vi "禹山叶绿素a校准.vi"() -> ()   [LabVIEW 2016, in "斯坦道多参数.lvlib"]
uses:
  <vilib>/Utility/miscctls.llb/LVPointTypeDef.ctl
  <vilib>/Analysis/NI_AALBase.lvlib
  <vilib>/Analysis/NI_AALPro.lvlib
  <vilib>/Utility/config.llb/NI_LVConfig.lvlib
panel:
  out "滤波设定":dbl
  out "通讯状态":string
  out "第二点校准值":dbl
  out "第一点校准值":dbl
  out "最小值":sgl format="%.2g"
  out "最大值":sgl format="%.2g"
  in  "校准停止":bool
  in  "校准模式":u16(ring) items=["两点校准", "单点校准"]
  in  "标液2":dbl
  in  "标液1":dbl
  out "波形图表":sgl(graph) caption="历史曲线"
  out "温度测量值":dbl caption="温度" format="%#.2f"
  out "变异系数":dbl format="%.6g"
  out "standard deviation":dbl caption="标准差" format="%0.2f"
  out "mean":dbl caption="均值" format="%0.2f"
  out "提示":string
  in  "校准启动":bool
  out "测试值":dbl format="%#.2f"
  out "电极斜率":dbl format="%#.6f"
  out "电极零点":dbl format="%#.6f"
  # "叶绿素a电极设定"
  # "请选择校准模式:"
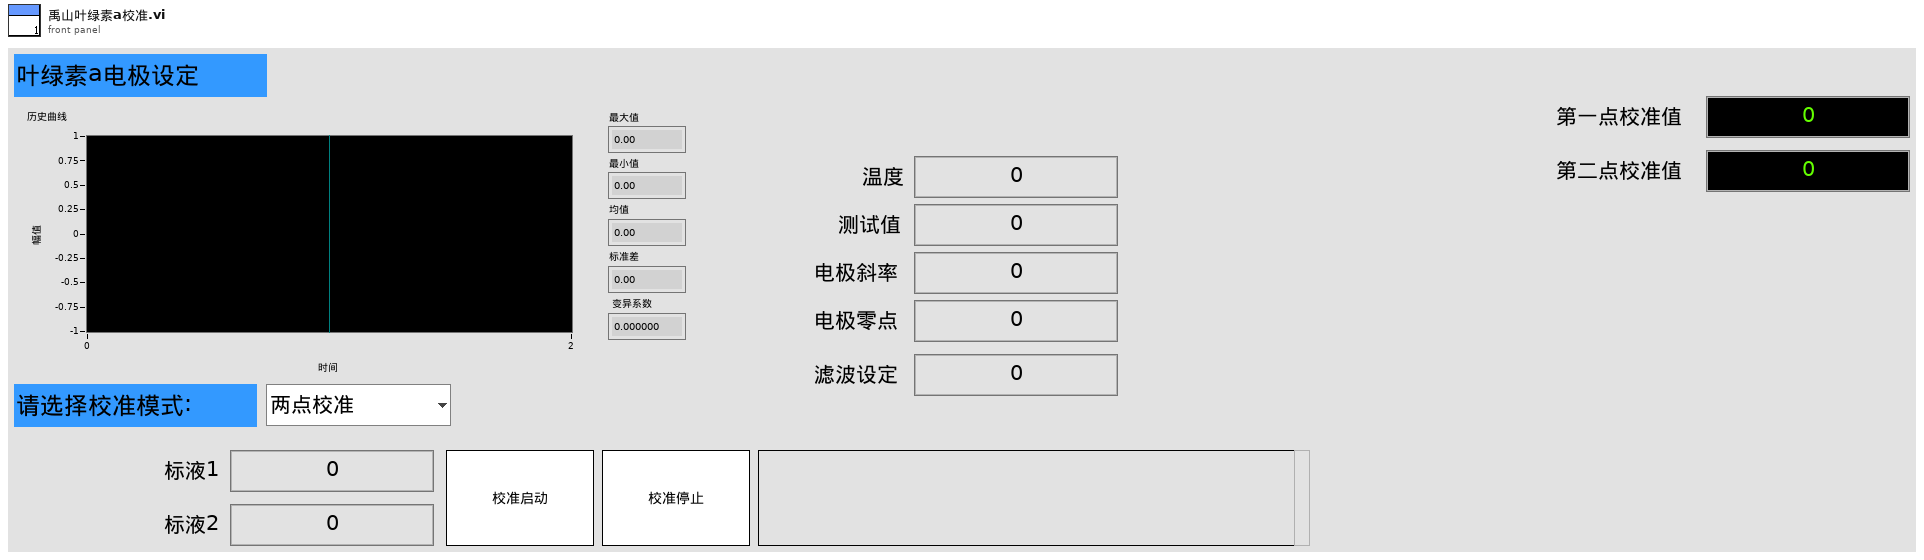
[diagram p1: front panel]
types:
  T1 = enum16{"pH", "DO", "Cond", "Turb", "ORP", "叶绿素a", "藻密度"}
  T2 = typedef "LVPointTypeDef.ctl" = cluster{"Horizontal":i16, "Vertical":i16}
  T3 = cluster{"pH":u32, "DO":u32, "Cond":u32, "Turb":u32, "叶绿素a":u32, "藻密度":u32, "ORP":u32}
  T4 = typedef "NI_LVConfig.lvlib/Config Data RefNum.ctl" = refnum<k1>
  T5 = enum8{"Enabled", "Disabled", "Disabled and Grayed Out"}
  T6 = cluster{"ph":bool, "DO":bool, "Cond":bool, "Turb":bool, "叶绿素a":bool, "藻密度":bool, "ORP":bool}
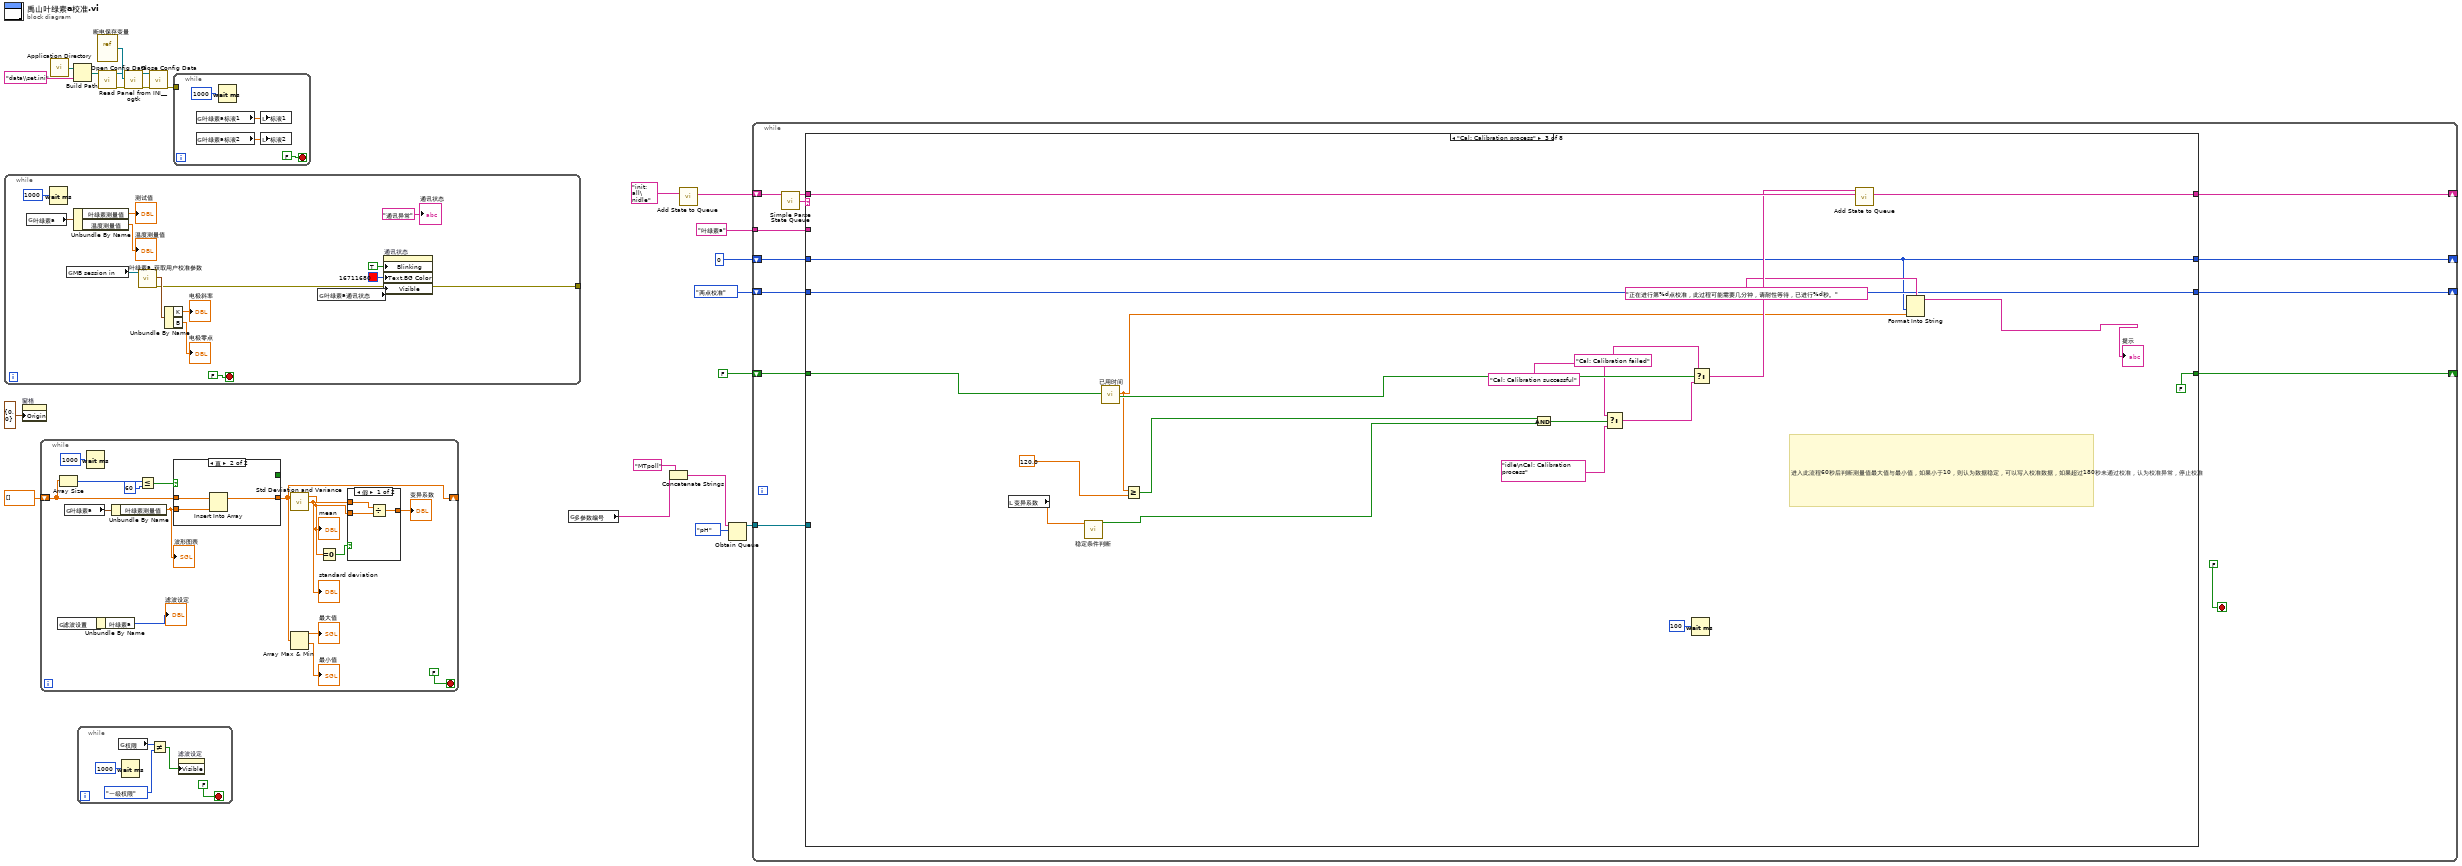
[diagram p0: block diagram]
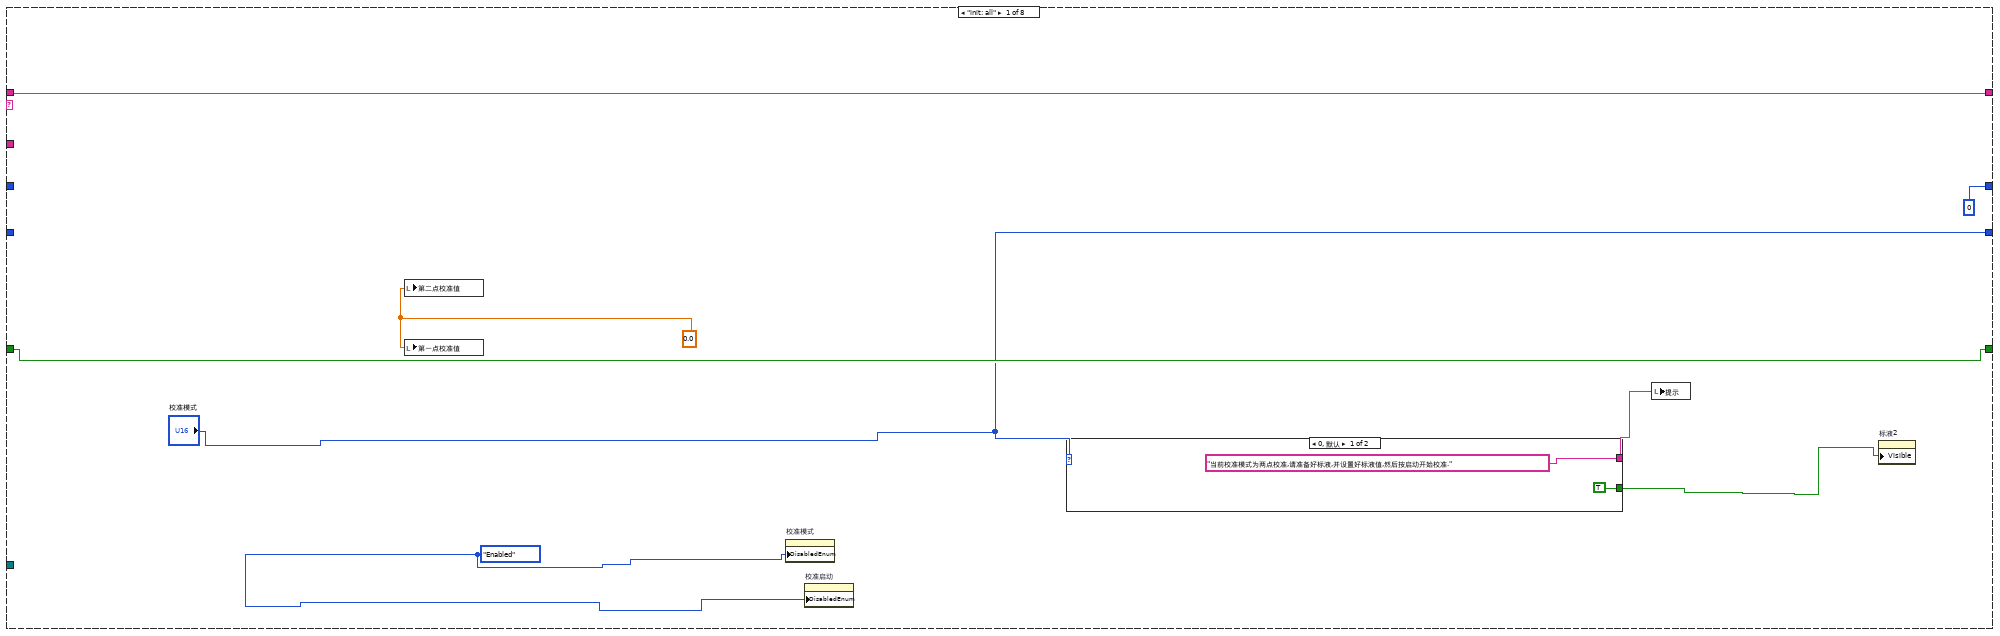
[diagram p2: hidden frame]
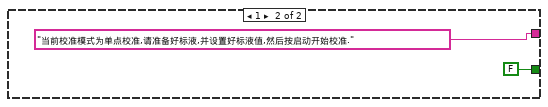
[diagram p3: hidden frame]
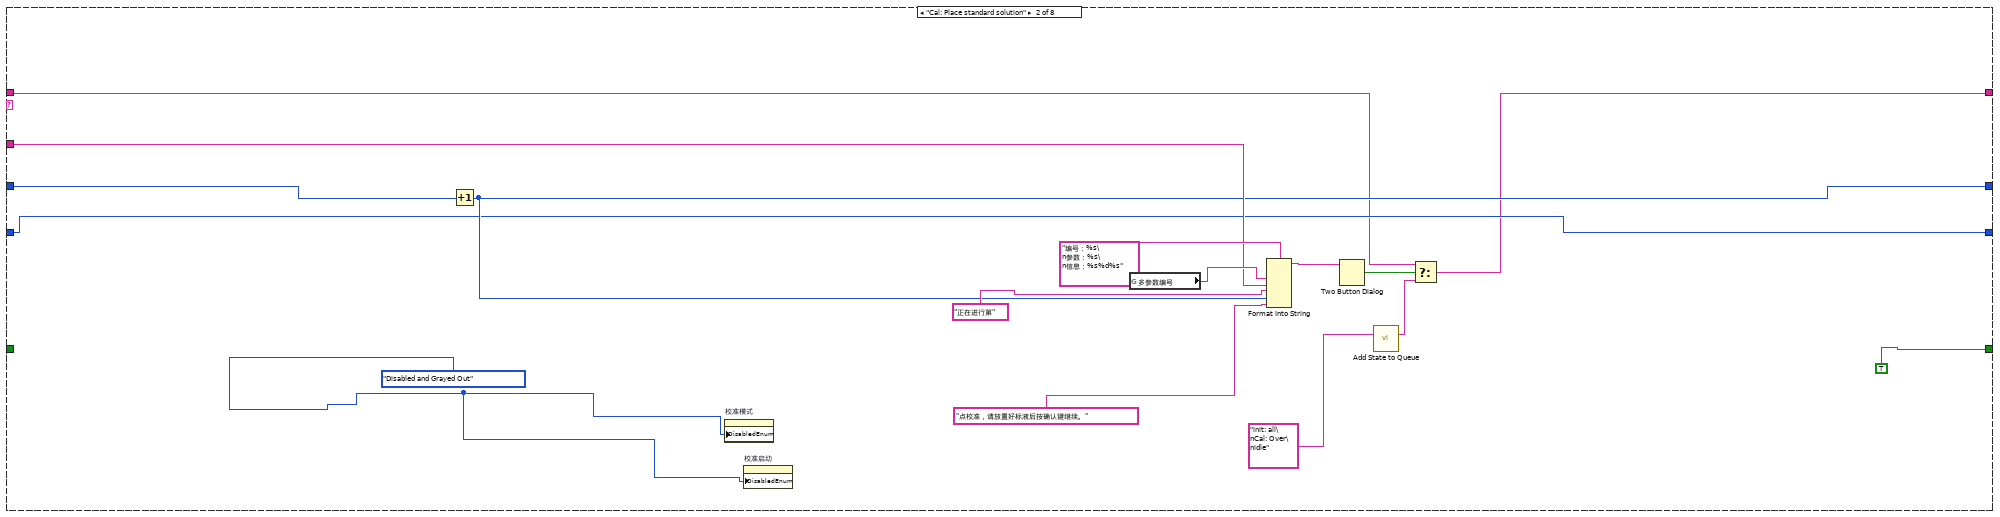
[diagram p4: hidden frame]
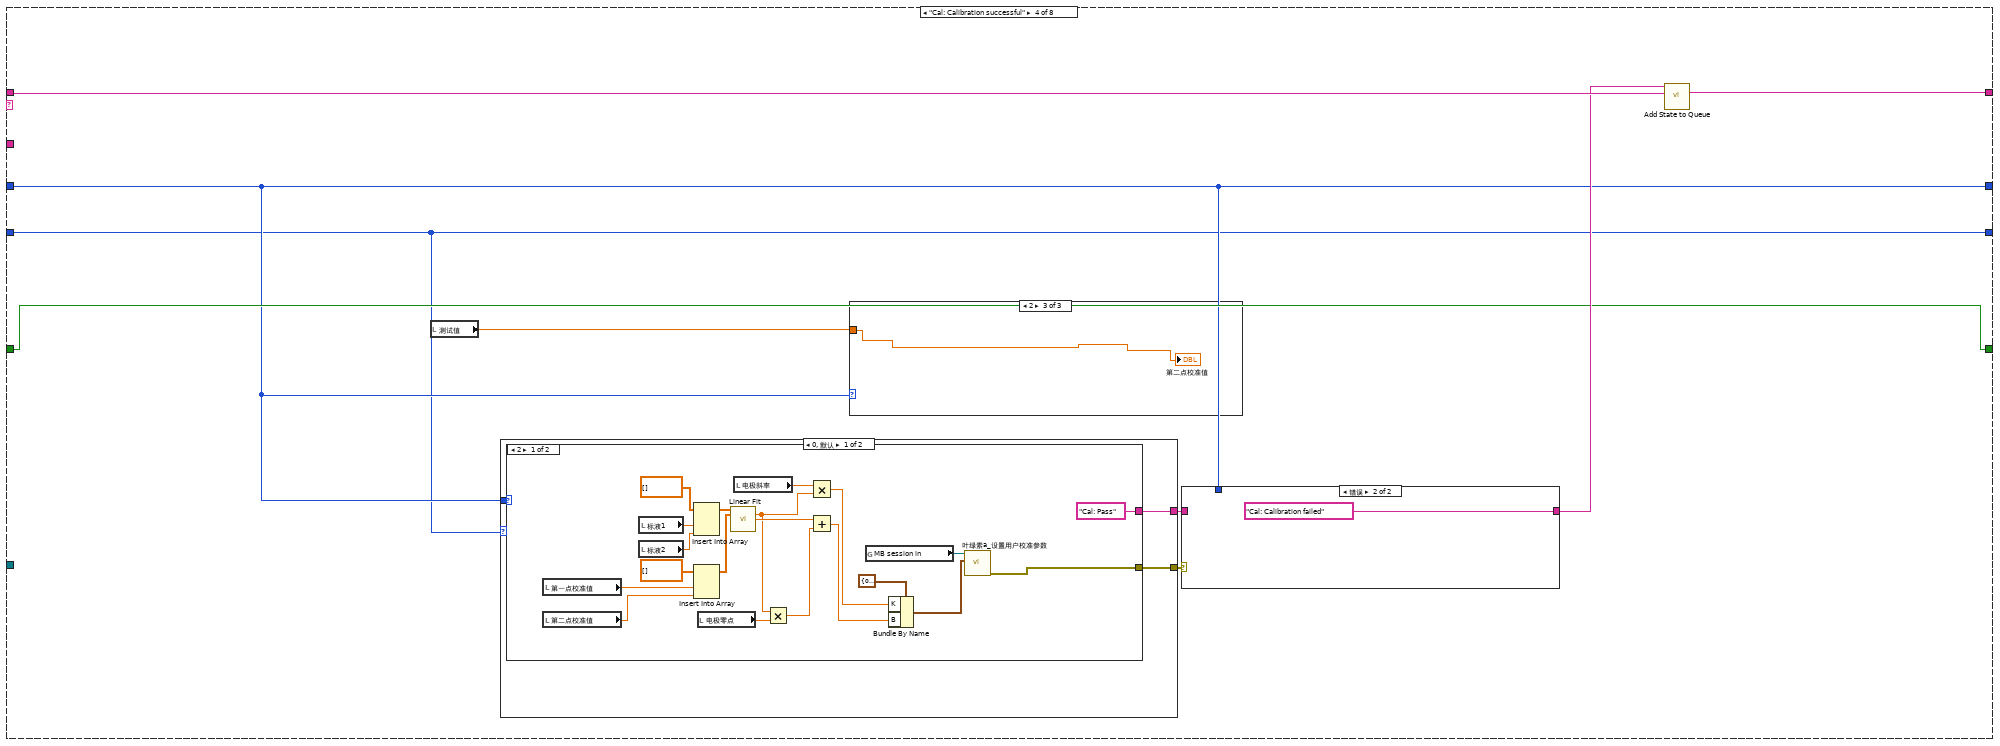
[diagram p5: hidden frame]
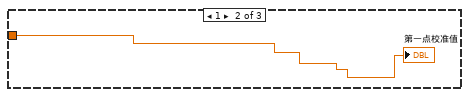
[diagram p7: hidden frame]
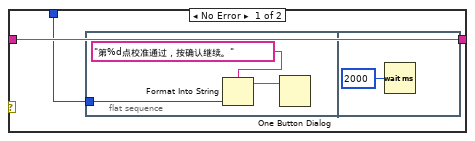
[diagram p8: hidden frame]
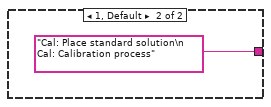
[diagram p9: hidden frame]
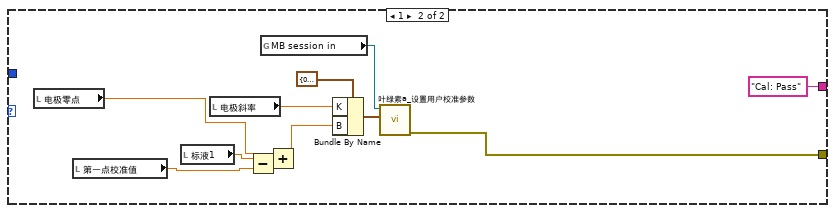
[diagram p10: hidden frame]
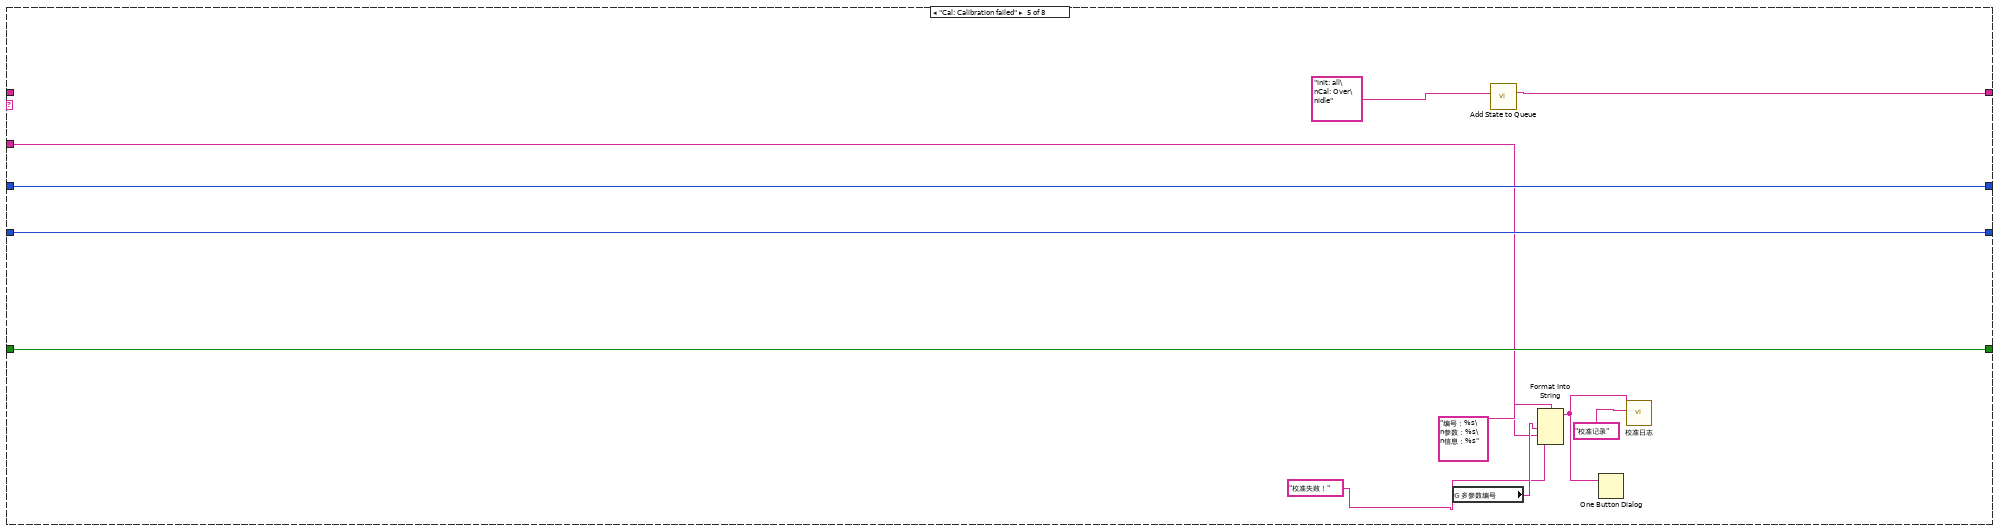
[diagram p11: hidden frame]
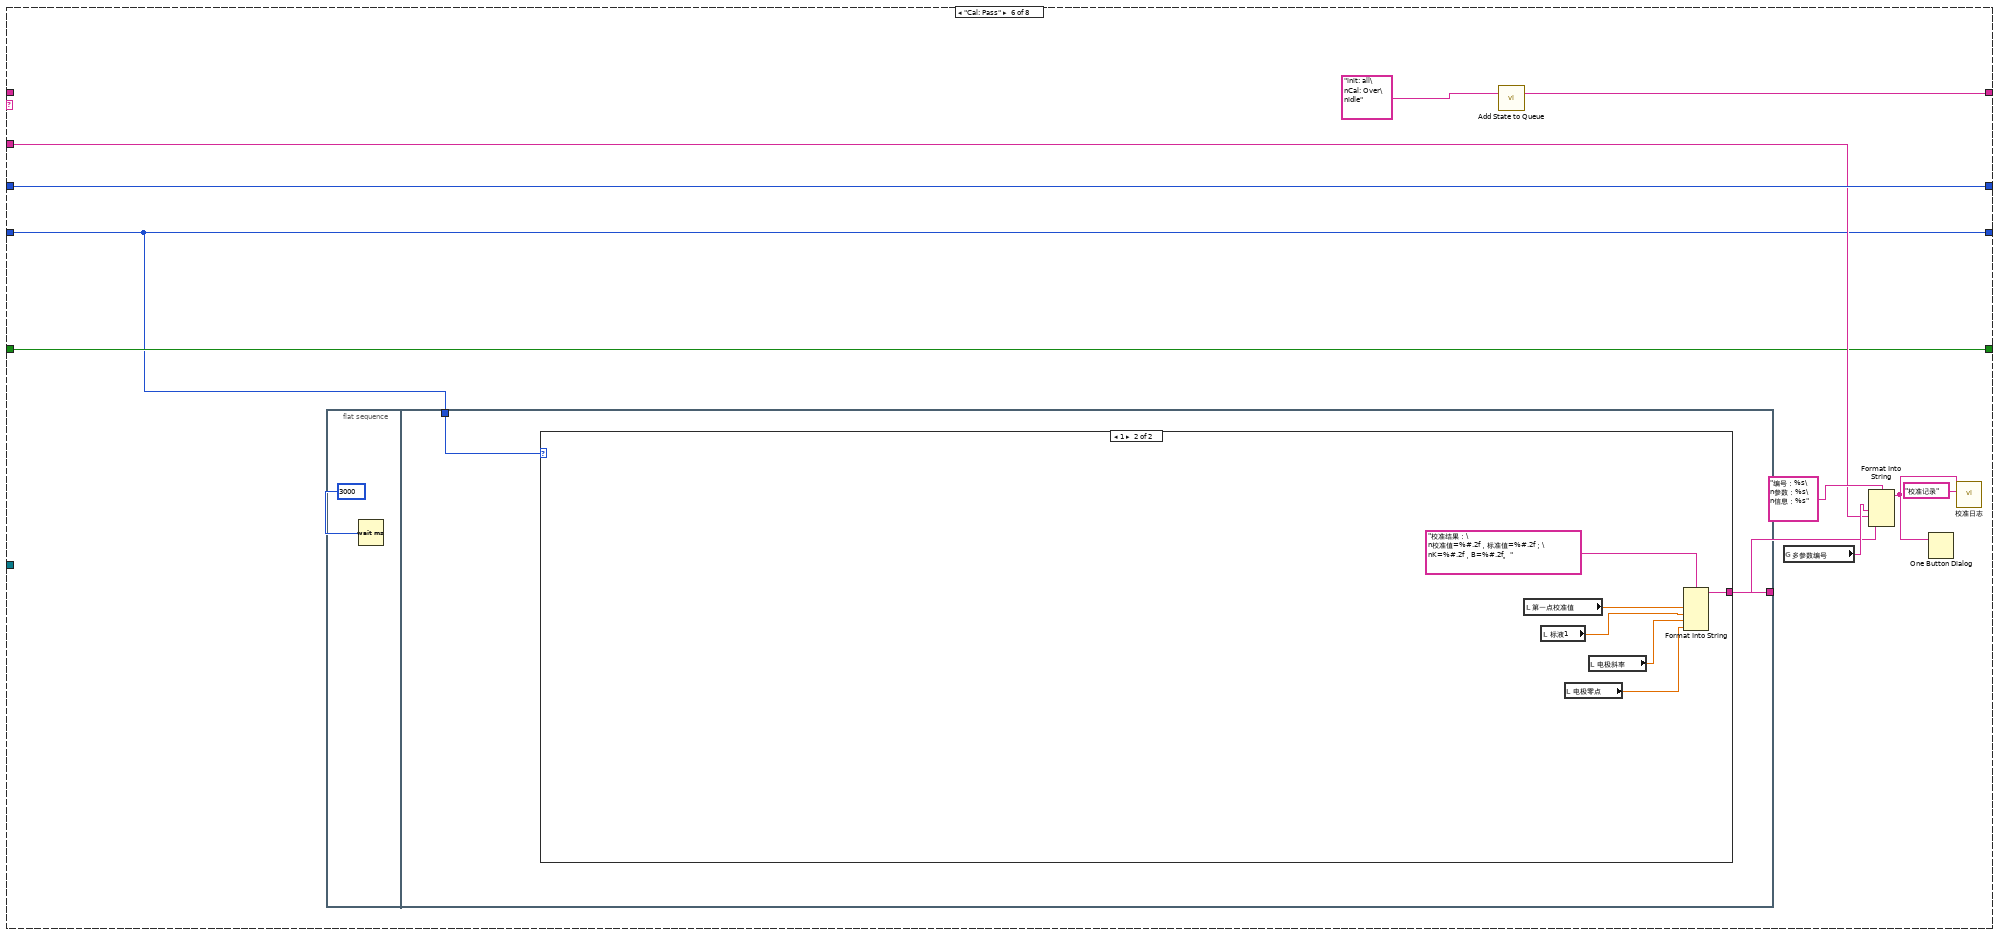
[diagram p12: hidden frame]
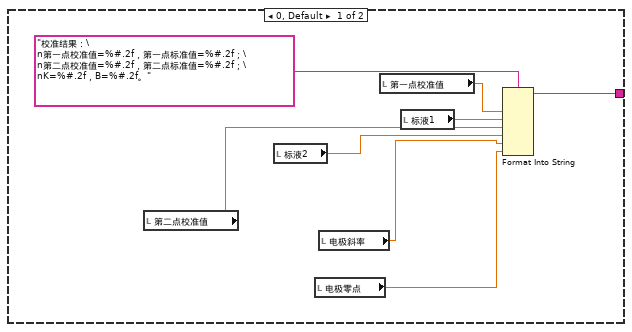
[diagram p13: hidden frame]
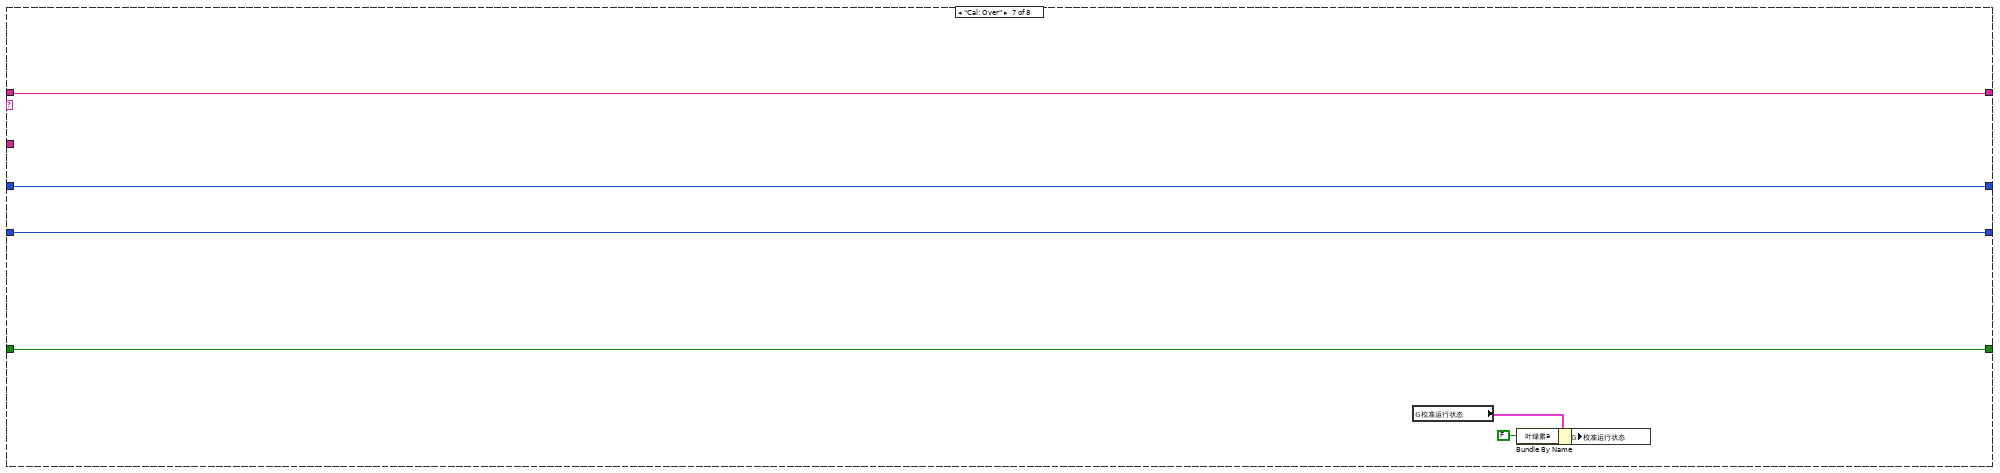
[diagram p14: hidden frame]
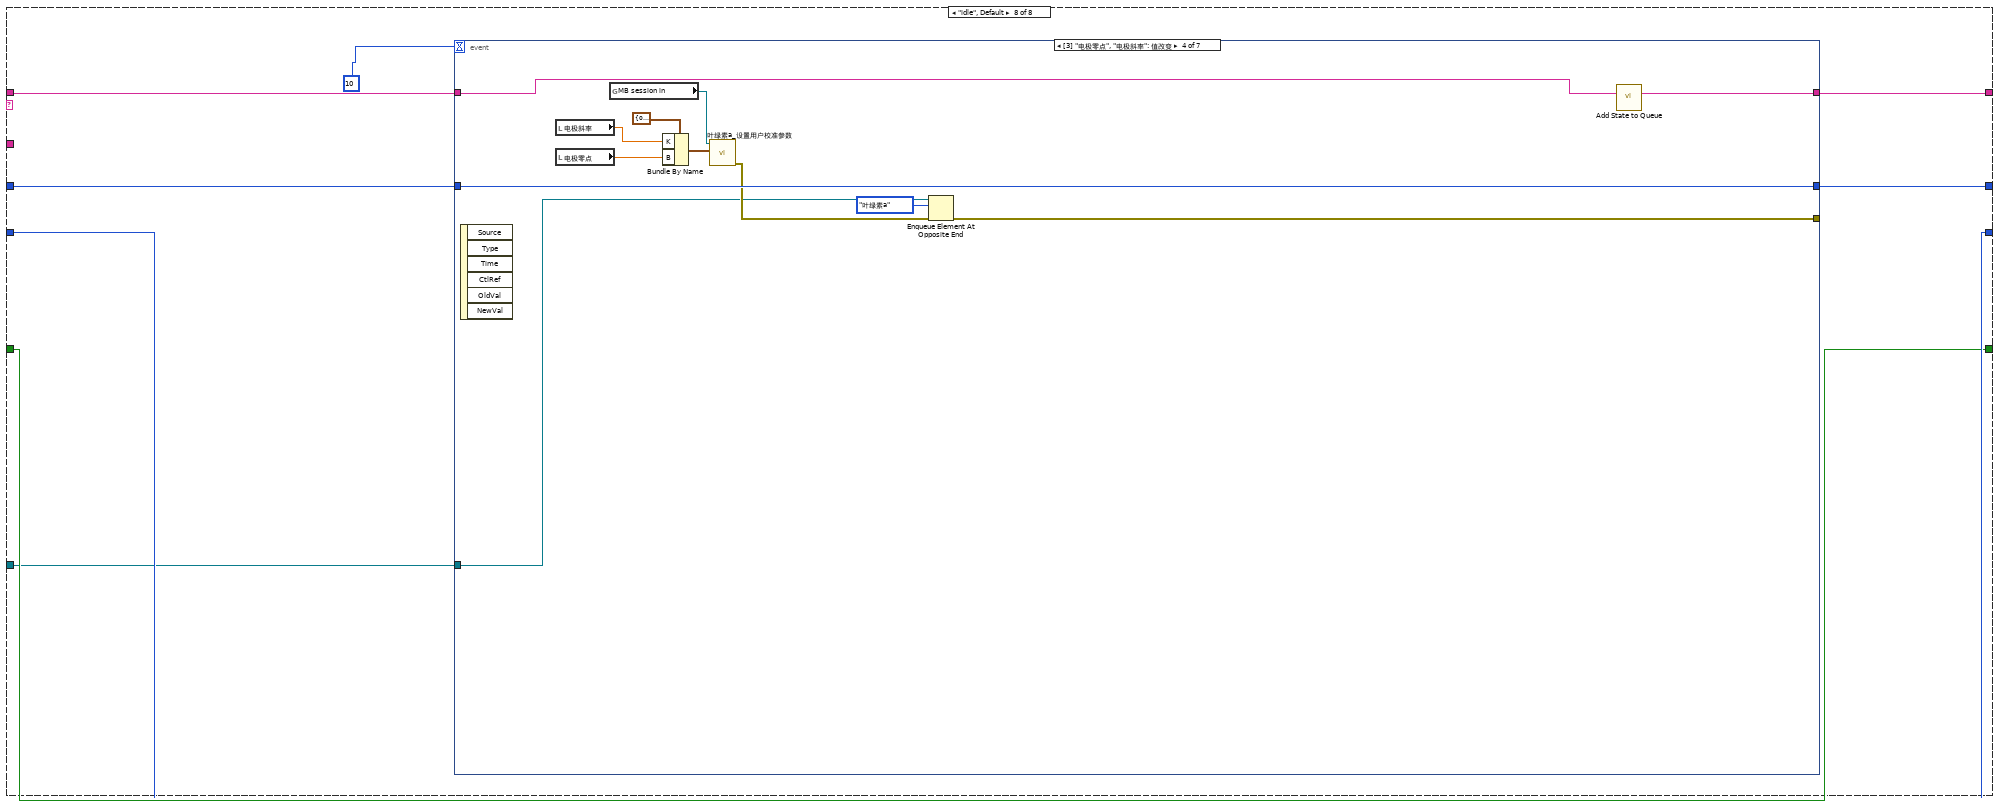
[diagram p15: hidden frame]
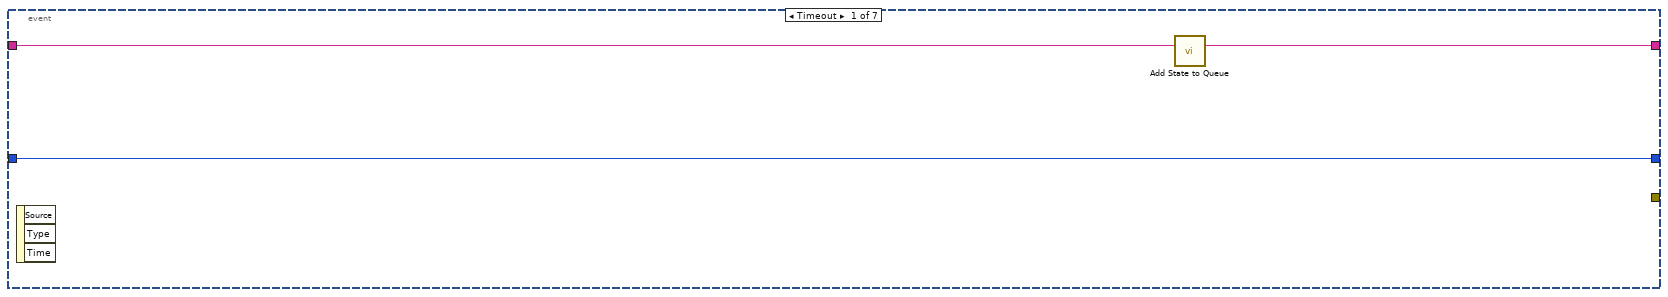
[diagram p16: hidden frame]
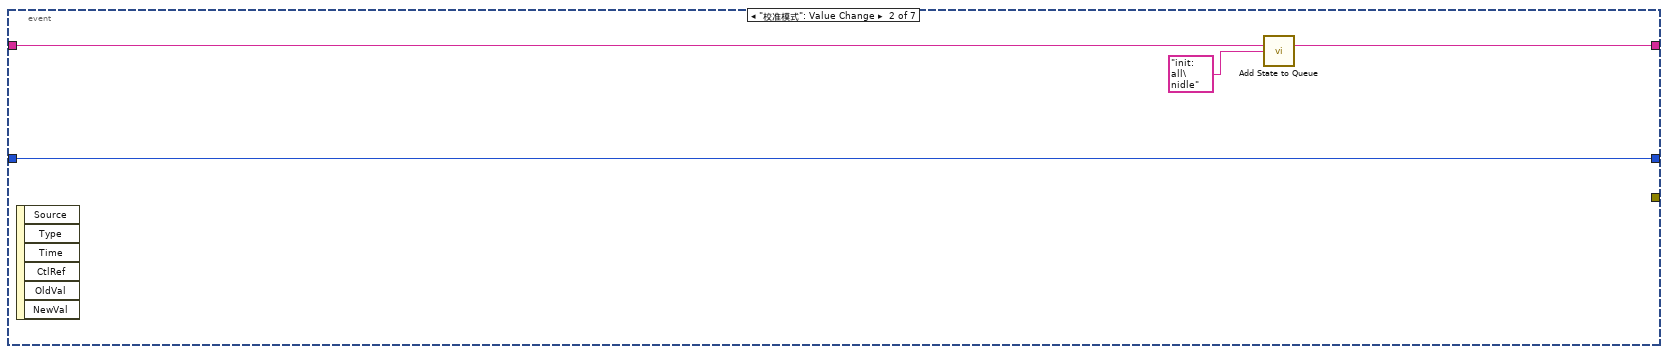
[diagram p17: hidden frame]
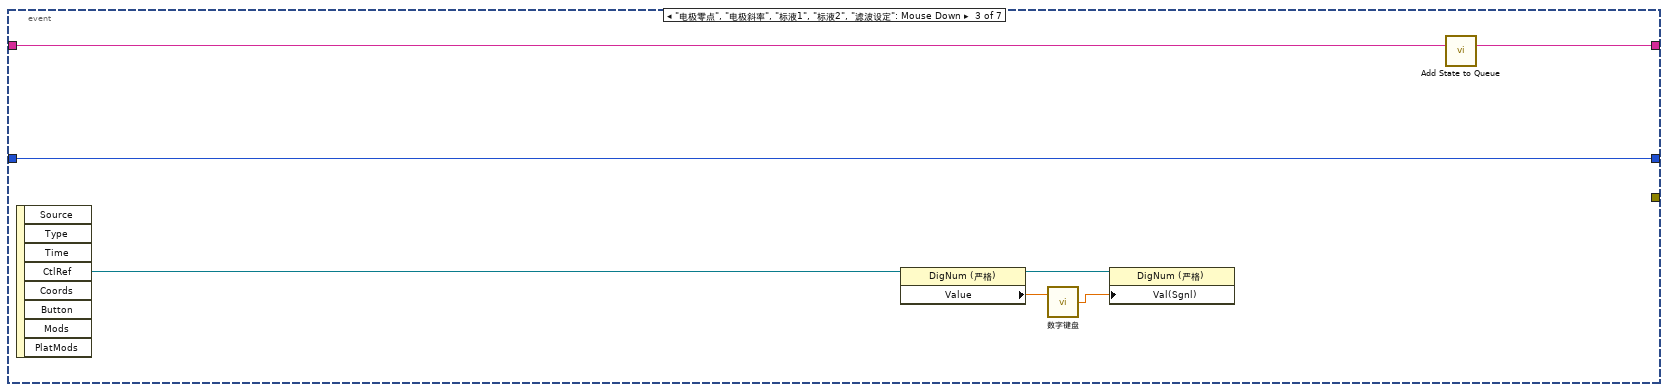
[diagram p18: hidden frame]
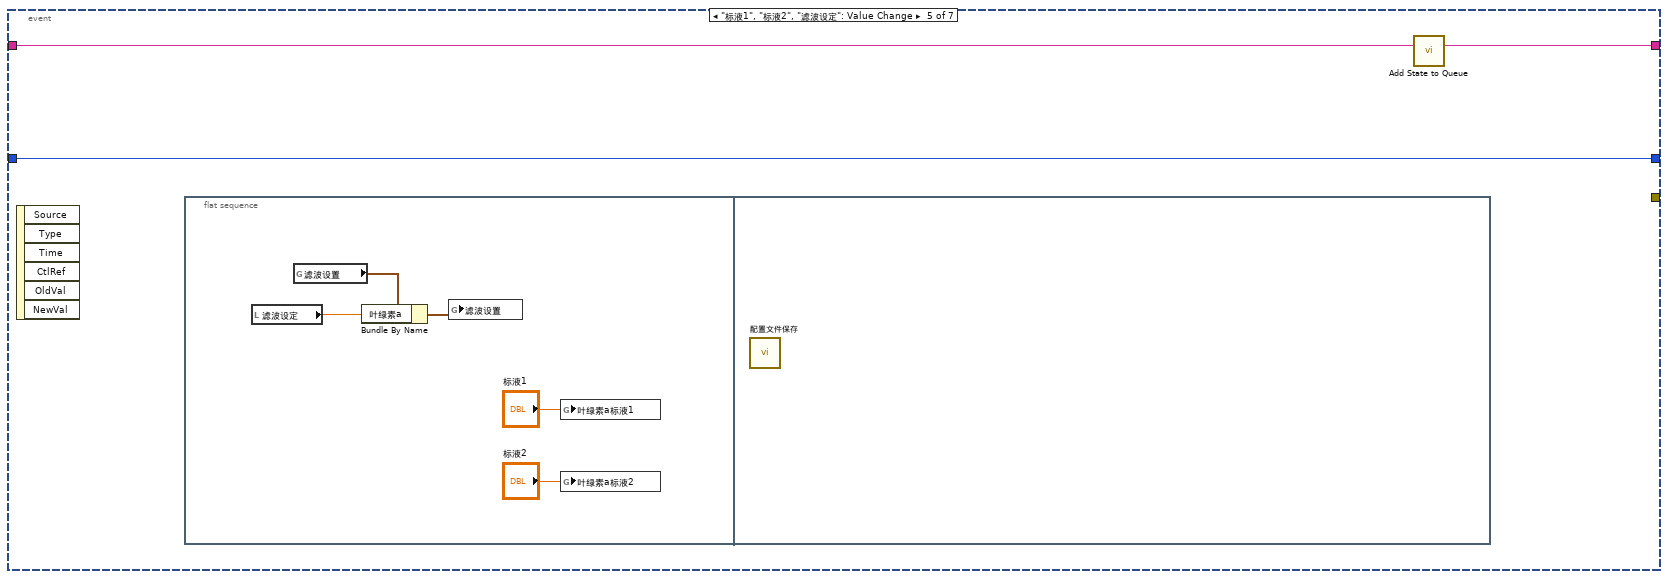
[diagram p19: hidden frame]
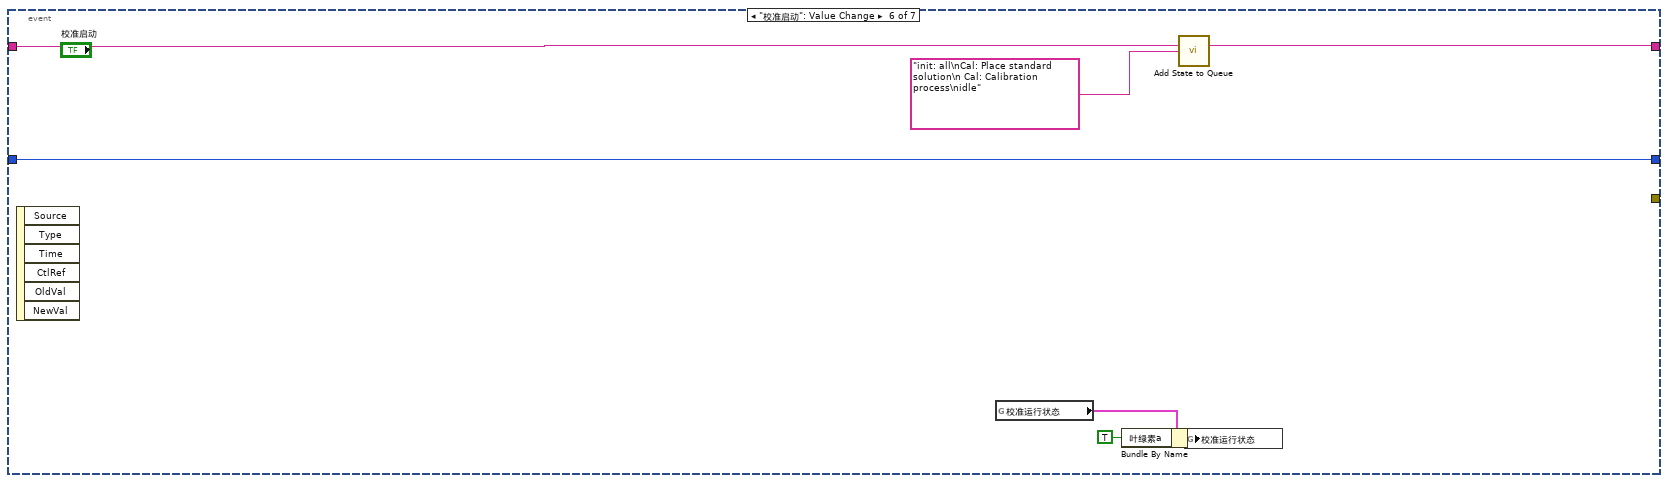
[diagram p20: hidden frame]
diagram:
  n1 = while {
    tunnel: [w31] -> _
    stop <- FALSE stop-if-true
    n2 = global read "禹山过程全局变量.vi" "叶绿素a"() -> (w28:cluster{"温度测量值":sgl, "叶绿素测量值":sgl, "错误标志":u16})
    n3 = Wait (ms)(milliseconds to wait=u32 1000 ("等待时间（毫秒）")) -> ()  [unwired: 1 out]
    n4 = global read "多参数全局变量.vi" "MB session in"() -> (w27:refnum<class "MB_Master.lvclass">)
    n5 = Unbundle By Name(w28) -> ("叶绿素测量值"=→"测试值":sgl, "温度测量值"=→"温度测量值":sgl)
    n6 = call "叶绿素a_获取用户校准参数.vi"("MB session in"=w27) -> ("error out"=w31:errorcluster, "输出值"=w34:cluster{"K":sgl, "B":sgl})  [unwired: 8 in, 1 out]
    n7 = Unbundle By Name(w34) -> ("K"=→"电极斜率":sgl, "B"=→"电极零点":sgl)
    n8 = global read "多参数全局变量.vi" "叶绿素a通讯状态"() -> (w23:bool)
    n9 = property on="通讯状态" class="Str"("Blinking"=TRUE ("闪烁"), "Text.BG Color"=u32 16711680, "Visible"=w23) -> ()  [unwired: 2 in, 2 out]
    "通讯状态" <- "通讯异常" ("当前串口")
  }
  n10 = property on="窗格" class="Pane"("Origin"=T2 {"Horizontal"=0, "Vertical"=0} ("原点")) -> ()  [unwired: 2 in, 2 out]
  n11 = while {
    shift-right: [w41] -> _
    shift-left: sgl[] [] -> [w49]
    stop <- FALSE stop-if-true
    n12 = global read "断电保存变量.vi" "滤波设置"() -> (w38:T3)
    n13 = Array Size(array=w49) -> (size(s)=w51:i32)
    n14 = global read "禹山过程全局变量.vi" "叶绿素a"() -> (w43:cluster{"温度测量值":sgl, "叶绿素测量值":sgl, "错误标志":u16})
    n15 = Wait (ms)(milliseconds to wait=u32 1000 ("等待时间（毫秒）")) -> ()  [unwired: 1 out]
    n16 = Unbundle By Name(w38) -> ("叶绿素a"=→"滤波设定":u32)
    n17 = Unbundle By Name(w43) -> ("叶绿素测量值"=w42:sgl)
    "波形图表" <- w42
    n18 = Less Or Equal?(x=w51, y=60) -> (x <= y?=w50:bool)
    n19 = case shown="真" w50 {
      tunnel: w49 -> [w62 w65]
      tunnel: w42 -> [w60 w64]
      tunnel: [w58 w63] -> w41
      tunnel: [TRUE _] -> _
      frame False {
        n20 = Replace Array Subset(array=w62, new element=w60) -> (w61:sgl[])  [unwired: 1 in]
        n21 = Rotate 1D Array(1:w61, 2:-1 ("n")) -> (0:w58:sgl[])
      }
      frame True {
        n22 = Insert Into Array(array=w65, new element=w64) -> (w63:sgl[])  [unwired: 1 in]
      }
    }
    n23 = call <vilib>:"Std Deviation and Variance.vi"("X"=w41) -> ("mean"=w44:dbl, "standard deviation"=w45:dbl)  [unwired: 1 in, 1 out]
    "standard deviation" <- w45
    "mean" <- w44
    n24 = Array Max & Min(array=w41) -> (max value=→"最大值":sgl, min value=→"最小值":sgl)  [unwired: 2 out]
    n25 = Equal To 0?(x=w44) -> (x = 0?=w48:bool)
    n26 = case shown="假" w48 {
      tunnel: w45 -> [w56 _]
      tunnel: [w55 _] -> w47
      tunnel: w44 -> [w54 _]
      frame False {
        n27 = Divide(x=w56, y=w54) -> (x/y=w55:dbl)
      }
      frame True {
      }
    }
    "变异系数" <- w47
  }
  n28 = call <vilib>:"Application Directory.vi"() -> ("Application Directory"=w17:path)
  n29 = Build Path(base path=w17, name or relative path="data\\set.ini" ("名称或相对路径")) -> (appended path=w18:path)
  n30 = while {
    stop <- FALSE stop-if-true
    n31 = global read "多参数全局变量.vi" "权限"() -> (w69:enum16{"一级权限", "二级权限", "三级权限"})
    n32 = Wait (ms)(milliseconds to wait=u32 1000 ("等待时间（毫秒）")) -> ()  [unwired: 1 out]
    n33 = Not Equal?(x=w69, y=enum16{"一级权限", "二级权限", "三级权限"}."一级权限") -> (x != y?=w66:bool)
    n34 = property on="滤波设定" class="DigNum (严格)"("Visible"=w66) -> ()  [unwired: 2 in, 2 out]
  }
  n35 = vi-ref "断电保存变量.vi"() -> (w20:refnum<vi>)
  n36 = call <vilib>:"Open Config Data.vi"("configuration file path"=w18) -> ("error out"=w14:errorcluster, "refnum"=w13:T4)  [unwired: 8 in, 1 out]
  n37 = call <userlib>:"Read Panel from INI__ogtk.vi"("error in (no error)"=w14, "VI ref"=w20, "refnum"=w13) -> ("error out"=w16:errorcluster, "refnum out"=w15:T4)  [unwired: 7 in]
  n38 = call <vilib>:"Close Config Data.vi"("error in (no error)"=w16, "refnum"=w15) -> ("error out"=w12:errorcluster)  [unwired: 8 in, 1 out]
  n39 = while {
    tunnel: w12 -> [_]
    stop <- FALSE stop-if-true
    n40 = global read "断电保存变量.vi" "叶绿素a标液1"() -> (w72:dbl)
    n41 = global read "断电保存变量.vi" "叶绿素a标液2"() -> (w71:dbl)
    n42 = Wait (ms)(milliseconds to wait=u32 1000 ("等待时间（毫秒）")) -> ()  [unwired: 1 out]
    n43 = local write "标液1"(w72) -> ()
    n44 = local write "标液2"(w71) -> ()
  }
  n45 = global read "多参数全局变量.vi" "多参数编号"() -> (w2:string)
  n46 = Concatenate Strings("MTpoll" ("名称（未命名）"), w2) -> (w4:string)
  n47 = call "Add State to Queue.vi"("State(s) In (\"\")"="init: all\nidle" ("State(s) In (\"\")")) -> ("States Out"=w10:string)  [unwired: 14 in]
  n48 = Obtain Queue(name (unnamed)=w4, element data type=T1."pH" ("枚举")) -> (queue out=w1:refnum<queue>)  [unwired: 3 in, 2 out]
  n49 = while {
    shift-right: [w83] -> _
    shift-left: w10 -> [w87]
    shift-right: [w80] -> _
    shift-left: 0 -> [w82]
    tunnel: "叶绿素a" ("State(s) In (\"\")") -> [w81]
    shift-right: [w78] -> _
    shift-left: enum16{"两点校准", "单点校准"}."两点校准" ("校准模式") -> [w79]
    shift-right: [w76] -> _
    shift-left: FALSE -> [w77]
    tunnel: w1 -> [w75]
    stop <- FALSE stop-if-true
    n50 = call "Simple Parse State Queue.vi"("State Queue"=w87) -> ("Remain States"=w84:string, "Next State"=w85:string)  [unwired: 13 in]
    n51 = case shown="\"Cal: Calibration process\"" w85 {
      tunnel: w84 -> [w95 w103 w135 w143 _ _ w235 w243]
      tunnel: [w95 w102 w134 w142 w197 w202 w235 w242] -> w83
      tunnel: w82 -> [_ w111 w120 w138 w200 w211 w234 w240]
      tunnel: w81 -> [_ w112 _ _ w191 w207 _ _]
      tunnel: [0 w109 w120 w138 w200 w211 w234 w241] -> w80
      tunnel: w79 -> [_ w108 w121 w137 w199 w203 w233 w239]
      tunnel: ["校准模式" w108 w121 w137 w199 w203 w233 w239] -> w78
      tunnel: w77 -> [w92 _ w123 w139 w198 w206 w232 w237]
      tunnel: [w92 TRUE FALSE w139 w198 w206 w232 w237] -> w76
      tunnel: w75 -> [_ _ _ _ _ _ _ w236]
      frame "init: all" {
        w89 = T5."Enabled" ("禁用")
        w91 = 0.0 ("第一点校准值")
        n52 = local write "第二点校准值"(w91) -> ()
        n53 = local write "第一点校准值"(w91) -> ()
        n54 = property on="校准模式" class="Ring (严格)"("DisabledEnum"=w89) -> ()  [unwired: 2 in, 2 out]
        n55 = property on="校准启动" class="Bool"("DisabledEnum"=w89) -> ()  [unwired: 2 in, 2 out]
        n56 = case shown="0, 默认" "校准模式" {
          tunnel: ["当前校准模式为两点校准,请准备好标液,并设置好标液值,然后按启动开始校准." ("提示") "当前校准模式为单点校准,请准备好标液,并设置好标液值,然后按启动开始校准." ("提示")] -> w94
          tunnel: [TRUE ("可见") FALSE ("可见")] -> w88
          frame 0, Default {
          }
          frame 1 {
          }
        }
        n57 = local write "提示"(w94) -> ()
        n58 = property on="标液2" class="DigNum (严格)"("Visible"=w88) -> ()  [unwired: 2 in, 2 out]
      }
      frame "Cal: Place standard solution" {
        w101 = T5."Disabled and Grayed Out" ("禁用")
        n59 = Increment(x=w111) -> (x+1=w109:i32)
        n60 = property on="校准模式" class="Ring (严格)"("DisabledEnum"=w101) -> ()  [unwired: 2 in, 2 out]
        n61 = property on="校准启动" class="Bool"("DisabledEnum"=w101) -> ()  [unwired: 2 in, 2 out]
        n62 = global read "多参数全局变量.vi" "多参数编号"() -> (w114:string)
        n63 = Format Into String(format string="编号：%s\n参数：%s\n信息：%s%d%s" ("格式字符串"), w114, w112, "正在进行第" ("消息"), w109, "点校准，请放置好标液后按确认键继续。" ("消息")) -> (resulting string=w106:string)  [unwired: 2 in, 1 out]
        n64 = Two Button Dialog(message=w106) -> (T button?=w105:bool)  [unwired: 2 in]
        n65 = call "Add State to Queue.vi"("State(s) In (\"\")"="init: all\nCal: Over\nidle" ("State(s) In (\"\")")) -> ("States Out"=w104:string)  [unwired: 14 in]
        n66 = Select(t=w103, s=w105, f=w104) -> (s? t:f=w102:string)
      }
      frame "Cal: Calibration process" {
        # "进入此流程60秒后判断测量值最大值与最小值，如果小于10，则认为数据稳定，可以写入校准数据，如果超过180秒未通过校准，认为校准异常，停止校准"
        n67 = local read "变异系数"() -> (w117:dbl)
        n68 = call "稳定条件判断.vi"("变异系数"=w117) -> ("布尔"=w116:bool)  [unwired: 10 in]
        n69 = call "已用时间"("Reset"=w123) -> ("Elapsed Time (s)"=w119:dbl, "Time has Elapsed"=w136:bool)  [unwired: 11 in, 6 out]
        n70 = Greater Or Equal?(x=w119, y=120.0) -> (x >= y?=w131:bool)
        n71 = And(x=w131, y=w116) -> (x .and. y?=w128:bool)
        n72 = Select(t="Cal: Calibration successful" ("State(s) In (\"\")"), s=w128, f="idle\nCal: Calibration process" ("State(s) In (\"\")")) -> (s? t:f=w127:string)
        n73 = Wait (ms)(milliseconds to wait=u32 100 ("等待时间（毫秒）")) -> ()  [unwired: 1 out]
        n74 = Select(t="Cal: Calibration failed" ("State(s) In (\"\")"), s=w136, f=w127) -> (s? t:f=w126:string)
        n75 = call "Add State to Queue.vi"("State(s) In Front (\"\")"=w126, "State(s) In (\"\")"=w135) -> ("States Out"=w134:string)  [unwired: 13 in]
        n76 = Format Into String(format string="正在进行第%d点校准，此过程可能需要几分钟，请耐性等待，已进行%d秒。" ("格式字符串"), w120, w119) -> (resulting string=→"提示":string)  [unwired: 2 in, 1 out]
      }
      frame "Cal: Calibration successful" {
        n77 = local read "测试值"() -> (w140:dbl)
        n78 = case shown="0, 默认" w137 {
          tunnel: [w157 w179] -> w145
          tunnel: [w156 "Cal: Pass" ("State(s) In (\"\")")] -> w144
          tunnel: w138 -> [w155 _]
          frame 0, Default {
            n79 = case shown="2" w155 {
              tunnel: [w158 _] -> w157
              tunnel: ["Cal: Pass" ("State(s) In (\"\")") "Cal: Place standard solution\n Cal: Calibration process" ("State(s) In (\"\")")] -> w156
              frame 2 {
                n80 = local read "第一点校准值"() -> (w160:dbl)
                n81 = local read "第二点校准值"() -> (w161:dbl)
                n82 = local read "标液1"() -> (w163:dbl)
                n83 = local read "标液2"() -> (w164:dbl)
                n84 = Insert Into Array(array=dbl[] [] ("Weight"), new element #1=w163, new element #2=w164) -> (w165:dbl[])  [unwired: 1 in]
                n85 = Insert Into Array(array=dbl[] [] ("Weight"), new element #1=w160, new element #2=w161) -> (w166:dbl[])  [unwired: 1 in]
                n86 = local read "电极零点"() -> (w172:dbl)
                n87 = call <vilib>:"Linear Fit.vi"("Y"=w165, "X"=w166) -> ("slope"=w173:dbl, "intercept"=w175:dbl)  [unwired: 9 in, 3 out]
                n88 = local read "电极斜率"() -> (w171:dbl)
                n89 = Multiply(x=w173, y=w172) -> (x*y=w174:dbl)
                n90 = Multiply(x=w171, y=w173) -> (x*y=w170:dbl)
                n91 = Add(x=w175, y=w174) -> (x+y=w176:dbl)
                n92 = global read "多参数全局变量.vi" "MB session in"() -> (w167:refnum<class "MB_Master.lvclass">)
                n93 = Bundle By Name(cluster=cluster{"K":sgl, "B":sgl} {"K"=0.0, "B"=0.0} ("用户校准参数"), "K"=w170, "B"=w176) -> (w168:cluster{"K":sgl, "B":sgl})
                n94 = call "叶绿素a_设置用户校准参数.vi"("用户校准参数"=w168, "MB session in"=w167) -> ("error out"=w158:errorcluster)  [unwired: 8 in, 1 out]
              }
              frame 1, Default {
              }
            }
          }
          frame 1 {
            n95 = local read "电极零点"() -> (w188:dbl)
            n96 = local read "第一点校准值"() -> (w184:dbl)
            n97 = local read "标液1"() -> (w185:dbl)
            n98 = local read "电极斜率"() -> (w183:dbl)
            n99 = Subtract(x=w185, y=w184) -> (x-y=w186:dbl)
            n100 = global read "多参数全局变量.vi" "MB session in"() -> (w180:refnum<class "MB_Master.lvclass">)
            n101 = Add(x=w188, y=w186) -> (x+y=w187:dbl)
            n102 = Bundle By Name(cluster=cluster{"K":sgl, "B":sgl} {"K"=0.0, "B"=0.0} ("用户校准参数"), "K"=w183, "B"=w187) -> (w181:cluster{"K":sgl, "B":sgl})
            n103 = call "叶绿素a_设置用户校准参数.vi"("用户校准参数"=w181, "MB session in"=w180) -> ("error out"=w179:errorcluster)  [unwired: 8 in, 1 out]
          }
        }
        n104 = case shown="2" w138 {
          tunnel: w140 -> [_ w146 w147]
          frame 0, Default {
          }
          frame 1 {
            "第一点校准值" <- w146
          }
          frame 2 {
            "第二点校准值" <- w147
          }
        }
        n105 = case shown="错误" w145 {
          tunnel: w144 -> [w149 _]
          tunnel: [w149 "Cal: Calibration failed" ("State(s) In (\"\")")] -> w141
          tunnel: w138 -> [w148 _]
          frame No Error {
            n106 = flat-sequence {
              tunnel: w148 -> [w150]
              frame #0 {
                n107 = Format Into String(format string="第%d点校准通过，按确认继续。" ("格式字符串"), w150) -> (resulting string=w152:string)  [unwired: 2 in, 1 out]
                n108 = One Button Dialog(message=w152) -> ()  [unwired: 1 in, 1 out]
              }
              frame #1 {
                n109 = Wait (ms)(milliseconds to wait=u32 2000 ("等待时间（毫秒）")) -> ()  [unwired: 1 out]
              }
            }
          }
          frame Error {
          }
        }
        n110 = call "Add State to Queue.vi"("State(s) In Front (\"\")"=w141, "State(s) In (\"\")"=w143) -> ("States Out"=w142:string)  [unwired: 13 in]
      }
      frame "Cal: Calibration failed" {
        n111 = global read "多参数全局变量.vi" "多参数编号"() -> (w194:string)
        n112 = call "Add State to Queue.vi"("State(s) In (\"\")"="init: all\nCal: Over\nidle" ("State(s) In (\"\")")) -> ("States Out"=w197:string)  [unwired: 14 in]
        n113 = Format Into String(format string="编号：%s\n参数：%s\n信息：%s" ("格式字符串"), w194, w191, "校准失败！" ("消息")) -> (resulting string=w193:string)  [unwired: 2 in, 1 out]
        n114 = One Button Dialog(message=w193) -> ()  [unwired: 1 in, 1 out]
        n115 = call "校准日志.vi"("table"="校准记录", "日志信息"=w193) -> ()  [unwired: 9 in, 1 out]
      }
      frame "Cal: Pass" {
        n116 = flat-sequence {
          tunnel: [w214] -> w204
          tunnel: w203 -> [w213]
          frame #0 {
            n117 = Wait (ms)(milliseconds to wait=u32 3000 ("等待时间（毫秒）")) -> ()  [unwired: 1 out]
          }
          frame #1 {
            n118 = case shown="1" w213 {
              tunnel: [w222 w228] -> w214
              frame 0, Default {
                n119 = local read "第二点校准值"() -> (w218:dbl)
                n120 = local read "标液2"() -> (w217:dbl)
                n121 = local read "电极零点"() -> (w215:dbl)
                n122 = local read "电极斜率"() -> (w216:dbl)
                n123 = local read "第一点校准值"() -> (w220:dbl)
                n124 = local read "标液1"() -> (w221:dbl)
                n125 = Format Into String(format string="校准结果：\n第一点校准值=%#.2f，第一点标准值=%#.2f；\n第二点校准值=%#.2f，第二点标准值=%#.2f；\nK=%#.2f，B=%#.2f。" ("提示"), w220, w221, w218, w217, w216, w215) -> (resulting string=w222:string)  [unwired: 2 in, 1 out]
              }
              frame 1 {
                n126 = local read "第一点校准值"() -> (w227:dbl)
                n127 = local read "标液1"() -> (w225:dbl)
                n128 = local read "电极零点"() -> (w223:dbl)
                n129 = local read "电极斜率"() -> (w224:dbl)
                n130 = Format Into String(format string="校准结果：\n校准值=%#.2f，标准值=%#.2f；\nK=%#.2f，B=%#.2f。" ("提示"), w227, w225, w224, w223) -> (resulting string=w228:string)  [unwired: 2 in, 1 out]
              }
            }
          }
        }
        n131 = call "Add State to Queue.vi"("State(s) In (\"\")"="init: all\nCal: Over\nidle" ("State(s) In (\"\")")) -> ("States Out"=w202:string)  [unwired: 14 in]
        n132 = global read "多参数全局变量.vi" "多参数编号"() -> (w208:string)
        n133 = Format Into String(format string="编号：%s\n参数：%s\n信息：%s" ("格式字符串"), w208, w207, w204) -> (resulting string=w205:string)  [unwired: 2 in, 1 out]
        n134 = One Button Dialog(message=w205) -> ()  [unwired: 1 in, 1 out]
        n135 = call "校准日志.vi"("table"="校准记录", "日志信息"=w205) -> ()  [unwired: 9 in, 1 out]
      }
      frame "Cal: Over" {
        n136 = global read "多参数全局变量.vi" "校准运行状态"() -> (w230:T6)
        n137 = Bundle By Name(cluster=w230, "叶绿素a"=FALSE) -> (w231:T6)
        n138 = global write "多参数全局变量.vi" "校准运行状态"(w231) -> ()
      }
      frame "idle", Default {
        n139 = event shown="[3] \"电极零点\", \"电极斜率\": 值改变" {
          selector: _ -> [_ _ _ _ _ _ _]
          dyn-events: _ -> [_ _ _ _ _ _ _]
          timeout: 10 -> [_ _ _ _ _ _ _]
          tunnel: [_ _ _ w260 _ _ _] -> _
          tunnel: w243 -> [w246 w250 w255 w261 w270 w284 _]
          tunnel: [w245 w249 w256 w268 w271 w283 w286] -> w242
          tunnel: [w244 w247 w257 w269 w272 w281 w287] -> w241
          tunnel: w240 -> [w244 w247 w257 w269 w272 w281 w287]
          tunnel: w236 -> [_ _ _ w259 _ _ _]
          event Timeout {
            n140 = event-data() -> ()  [unwired: 1 in, 3 out]
            n141 = call "Add State to Queue.vi"("State(s) In (\"\")"=w246) -> ("States Out"=w245:string)  [unwired: 14 in]
          }
          event "校准模式": Value Change {
            n142 = event-data() -> ()  [unwired: 1 in, 6 out]
            n143 = call "Add State to Queue.vi"("State(s) In (\"\")"=w250, "State(s) At Back (\"\")"="init: all\nidle" ("State(s) In (\"\")")) -> ("States Out"=w249:string)  [unwired: 13 in]
          }
          event "电极零点", "电极斜率", "标液1", "标液2", "滤波设定": Mouse Down {
            n144 = event-data() -> ("CtlRef"=w254:refnum<vi>)  [unwired: 1 in, 7 out]
            n145 = property class="DigNum (严格)"(reference=w254) -> (reference out=w251:refnum<vi>, "Value"=w252:dbl)  [unwired: 1 in, 1 out]
            n146 = call "数字键盘.vi"("OldNumber"=w252) -> ("NewNumber"=w253:dbl)  [unwired: 1 in]
            n147 = property class="DigNum (严格)"(reference=w251, "Val(Sgnl)"=w253) -> ()  [unwired: 1 in, 2 out]
            n148 = call "Add State to Queue.vi"("State(s) In (\"\")"=w255) -> ("States Out"=w256:string)  [unwired: 14 in]
          }
          event "电极零点", "电极斜率": Value Change {
            n149 = event-data() -> ()  [unwired: 1 in, 6 out]
            n150 = local read "电极斜率"() -> (w265:dbl)
            n151 = local read "电极零点"() -> (w264:dbl)
            n152 = global read "多参数全局变量.vi" "MB session in"() -> (w263:refnum<class "MB_Master.lvclass">)
            n153 = Bundle By Name(cluster=cluster{"K":sgl, "B":sgl} {"K"=0.0, "B"=0.0} ("用户校准参数"), "K"=w265, "B"=w264) -> (w266:cluster{"K":sgl, "B":sgl})
            n154 = call "叶绿素a_设置用户校准参数.vi"("用户校准参数"=w266, "MB session in"=w263) -> ("error out"=w262:errorcluster)  [unwired: 8 in, 1 out]
            n155 = Enqueue Element At Opposite End(queue=w259, element=T1."叶绿素a" ("元素"), error in (no error)=w262) -> (error out=w260:errorcluster)  [unwired: 1 in, 2 out]
            n156 = call "Add State to Queue.vi"("State(s) In (\"\")"=w261) -> ("States Out"=w268:string)  [unwired: 14 in]
          }
          event "标液1", "标液2", "滤波设定": Value Change {
            n157 = event-data() -> ()  [unwired: 1 in, 6 out]
            n158 = flat-sequence {
              frame #0 {
                n159 = local read "滤波设定"() -> (w273:dbl)
                n160 = global read "断电保存变量.vi" "滤波设置"() -> (w275:T3)
                n161 = Bundle By Name(cluster=w275, "叶绿素a"=w273) -> (w274:T3)
                n162 = global write "断电保存变量.vi" "滤波设置"(w274) -> ()
                n163 = global write "断电保存变量.vi" "叶绿素a标液1"("标液1") -> ()
                n164 = global write "断电保存变量.vi" "叶绿素a标液2"("标液2") -> ()
              }
              frame #1 {
                n165 = call "配置文件保存.vi"() -> ()  [unwired: 12 in]
              }
            }
            n166 = call "Add State to Queue.vi"("State(s) In (\"\")"=w270) -> ("States Out"=w271:string)  [unwired: 14 in]
          }
          event "校准启动": Value Change {
            n167 = event-data() -> ()  [unwired: 1 in, 6 out]
            n168 = global read "多参数全局变量.vi" "校准运行状态"() -> (w279:T6)
            n169 = Bundle By Name(cluster=w279, "叶绿素a"=TRUE) -> (w280:T6)
            n170 = call "Add State to Queue.vi"("State(s) In (\"\")"=w284, "State(s) At Back (\"\")"="init: all\nCal: Place standard solution\n Cal: Calibration process\nidle" ("State(s) In (\"\")")) -> ("States Out"=w283:string)  [unwired: 13 in]
            n171 = global write "多参数全局变量.vi" "校准运行状态"(w280) -> ()
          }
          event "校准停止": Value Change {
            n172 = event-data() -> ()  [unwired: 1 in, 6 out]
            n173 = call "Add State to Queue.vi"("State(s) In (\"\")"="init: all\nCal: Over\nidle" ("State(s) In (\"\")")) -> ("States Out"=w286:string)  [unwired: 14 in]
          }
        }
      }
    }
  }
